vi "字符串操作函数（四）.vi"() -> ()   [LabVIEW 2010]
panel:
  out "输出":dbl
  out "剩余字符串":string
  out "输出3":string
  out "输出2":dbl
  out "输出1":string
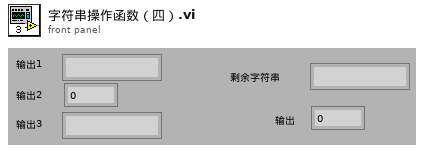
[diagram p1: front panel]
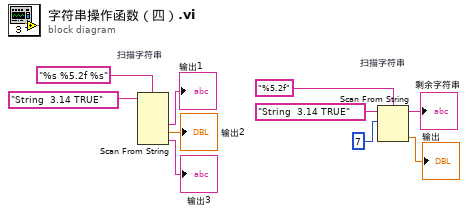
[diagram p0: block diagram]
diagram:
  n1 = Scan From String "扫描字符串"(format string="%s %5.2f %s", input string="String  3.14 TRUE" ("格式化输出字符串")) -> (output 1=→"输出1":string, output 2=→"输出2":dbl, output 3=→"输出3":string)  [unwired: 5 in, 3 out]
  n2 = Scan From String "扫描字符串"(format string="%5.2f", input string="String  3.14 TRUE" ("格式化输出字符串"), initial scan location=u32 7) -> (remaining string=→"剩余字符串":string, output 1=→"输出":dbl)  [unwired: 2 in, 2 out]
